vi "Detect_circles.vi"() -> ()   [LabVIEW 2020]
uses:
  <vilib>/vision/NI_Vision_Development_Module.lvlib
panel:
  out "error out":errorcluster
  out "Circles":T1(array[cluster]) {"Position"."Y" format="%.2f"; "Position"."X" format="%.2f"}
  in  "error_in":errorcluster
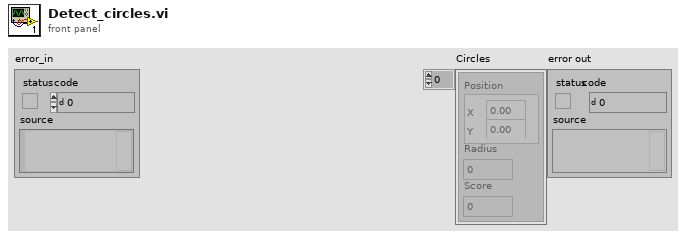
[diagram p1: front panel]
types:
  T1 = cluster{"Position":cluster{"X":sgl, "Y":sgl}, "Radius":dbl, "Score":dbl}[]
  T2 = typedef "IMAQ Image.ctl" = refnum<image>
  T3 = typedef "Image_Cluster.ctl" = cluster{"Detector_info":cluster{"No. of detectors":dbl, "Detector_Array":string[][]}, "Corner_info":cluster{"Corner_Array":dbl[][]}, "ROI":cluster{"Corners":cluster{"Global Rectangle":i32[], "Contours":cluster{"ID":enum32{"External", "Internal"}, "Type":u32, "Coordinates":i32[]}[]}[], "Detectors":cluster{"Global Rectangle":i32[], "Contours":cluster{"ID":enum32{"External", "Internal"}, "Type":u32, "Coordinates":i32[]}[]}[]}, "Shape_Detect":cluster{"Match_score":dbl, "Curve Parameters":T4, "Match Options":T5, "Circle Descriptor":cluster{"Min Radius":dbl, "Max Radius":dbl}}, "Path":cluster{"Config":path, "Map":path}}
  T4 = typedef "IMAQ Curve Parameters.ctl" = cluster{"Extraction Mode":u32, "Edge Threshold":i32, "Edge Filter Size":u32, "Min Length":i32, "Row Search Step Size":i32, "Col Search Step Size":i32, "Max Endpoint Gap":i32, "Closed":bool, "Subpixel":bool}
  T5 = typedef "ShapeDetectionMatchOptions.ctl" = cluster{"Rotation":bool, "Scale":bool, "Occlusion":bool, "Range Settings":T6[]}
  T6 = typedef "IMAQ Match Range Setting.ctl" = cluster{"Match Constraints":u32, "Min":dbl, "Max":dbl}
  T7 = cluster{"Global Rectangle":i32[], "Contours":cluster{"ID":enum32{"External", "Internal"}, "Type":u32, "Coordinates":i32[]}[]}[]
  T8 = cluster{"Global Rectangle":i32[], "Contours":cluster{"ID":enum32{"External", "Internal"}, "Type":u32, "Coordinates":i32[]}[]}
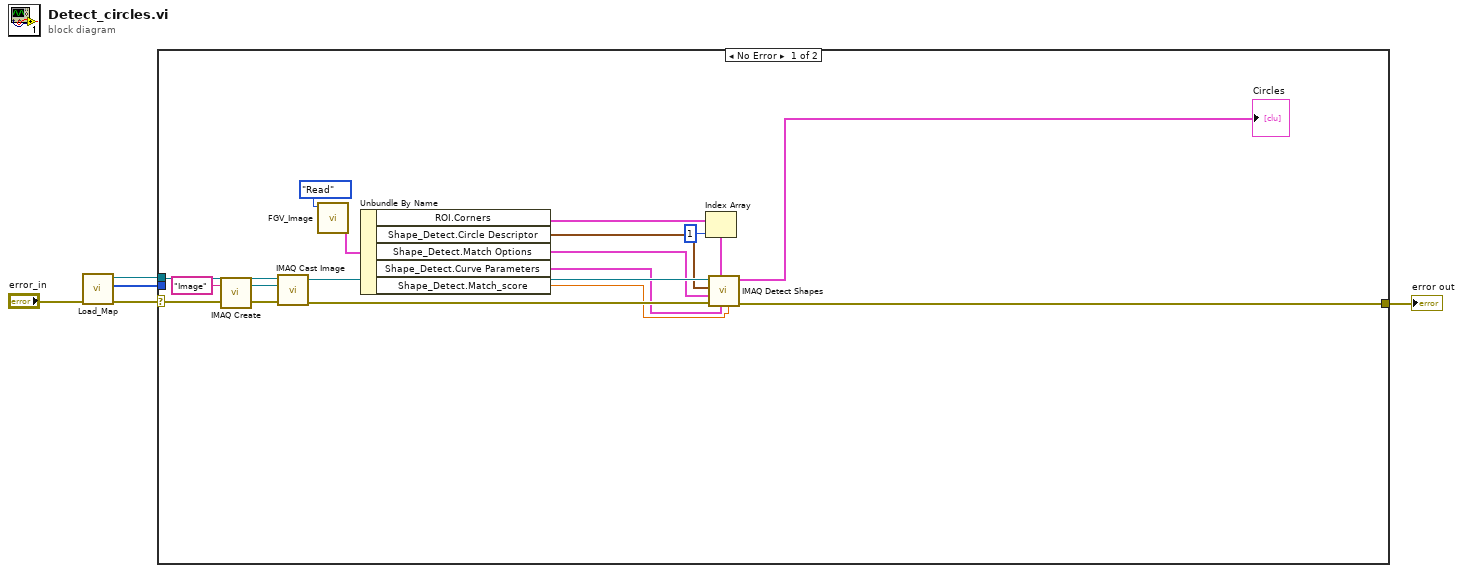
[diagram p0: block diagram]
diagram:
  n1 = call "Load_Map.vi"("error in (no error)"="error_in") -> ("error out"=w4:errorcluster, "image size"=w2:i32[], "Image Out"=w3:T2)  [unwired: 7 in]
  n2 = case shown="No Error" w4 {
    selector: w4 -> [w19 w24]
    tunnel: w3 -> [w22 _]
    tunnel: w2 -> [_ _]
    tunnel: [w15 w24] -> w1
    frame No Error {
      n3 = call "IMAQ Create"("Image Name"="Image", "error in (no error)"=w19) -> ("New Image"=w17:T2, "error out"=w18:errorcluster)  [unwired: 3 in]
      n4 = call "IMAQ Cast Image"("error in (no error)"=w18, "Image Dst"=w17, "Image Src"=w22) -> ("error out"=w20:errorcluster, "Image Dst Out"=w21:T2)  [unwired: 7 in]
      n5 = call "FGV_Image.vi"("Action"=enum16{"Read", "Write", ""}."Read") -> ("Image_Cluster_out"=w13:T3)  [unwired: 10 in]
      n6 = Unbundle By Name(w13) -> ("ROI.Corners"=w12:T7, "Shape_Detect.Circle Descriptor"=w10:cluster{"Min Radius":dbl, "Max Radius":dbl}, "Shape_Detect.Match Options"=w9:T5, "Shape_Detect.Curve Parameters"=w8:T4, "Shape_Detect.Match_score"=w7:dbl)
      n7 = Index Array(array=w12, index=1) -> (element=w11:T8)
      n8 = call-poly "IMAQ Detect Shapes"("Minimum match score"=w7, "Curve Parameters"=w8, "ROI Descriptor"=w11, "error in (no error)"=w20, "Match Options"=w9, "Circle Descriptor"=w10, "Image"=w21) -> ("error out"=w15:errorcluster, "Circles"=→"Circles":T1)  [unwired: 2 in, 1 out]
    }
    frame Error {
    }
  }
  "error out" <- w1
